vi "Actor Core.vi"(8 "error in":errorcluster, 11 "SongQueueActor in":refnum<class "SongQueueActor.lvclass">) -> (0 "error out":errorcluster, 3 "Actor out":refnum<class "Actor.lvclass">)   [LabVIEW 2015, in "SongQueueActor.lvlib" / "SongQueueActor.lvclass"]
doc: "(<B>Filename</B>: Actor Framework.lvlib:Actor.lvclass:Actor Core.vi)\n\nReceives messages to the actor, reacts to them, and initiates any error handling that may shut the actor down.\n\nDescendant classes may override this VI to append parallel tasks for the actor to complete while it handles messages. Overrides use the Call Parent Method node."
uses:
  SongQueueActor.lvclass
  <vilib>/ActorFramework/Actor/Actor.lvclass
  builds/xctls/Song Queue/Song Queue.lvlibp/app/xctls/SongQueue/Song Queue.xctl
  SongPlayerActor/SongPlayerActor/SongPlayerActor.lvclass
  builds/xctls/Song Queue/Song Queue.lvlibp/app/controls/Queue Song Display.ctl
  builds/xctls/Song Queue/Song Queue.lvlibp/file/MusicElement/Song/Song Duration.ctl
  builds/xctls/Song Queue/Song Queue.lvlibp/app/controls/Dequeue Control.ctl
  SongQueueActor.lvclass/SongQueueActor.ctl
  <vilib>/ActorFramework/Actor/Actor.lvclass/Actor.ctl
  <vilib>/ActorFramework/Message Enqueuer/Message Enqueuer.lvclass/Message Enqueuer.ctl
  <vilib>/ActorFramework/Message Enqueuer/Init from Existing Queue.vi
  <vilib>/ActorFramework/Message Enqueuer/Enqueue.vi
  <vilib>/ActorFramework/Message Priority Queue/Priority Enqueue.vi
  <vilib>/ActorFramework/Message Enqueuer/Message Enqueuer.lvclass
  <vilib>/ActorFramework/Stop Msg/Stop Msg.lvclass
  SongPlayerActor/SongPlayerActor Messages/Embed Actor Core In Subpanel Msg/Embed Actor Core In Subpanel Msg.lvclass
  builds/xctls/Song Queue/Song Queue.lvlibp
  builds/xctls/Song Queue/Song Queue.lvlibp/file/MusicElement/Song/Song.lvclass
  SongQueueActor Messages/Remove Song From Queue by Index Msg/Remove Song From Queue by Index Msg.lvclass
panel:
  in  "UI Tabs":enum32{"Main", "Debug"}(tab)
  in  "Song Queue":T1[](xcontrol)
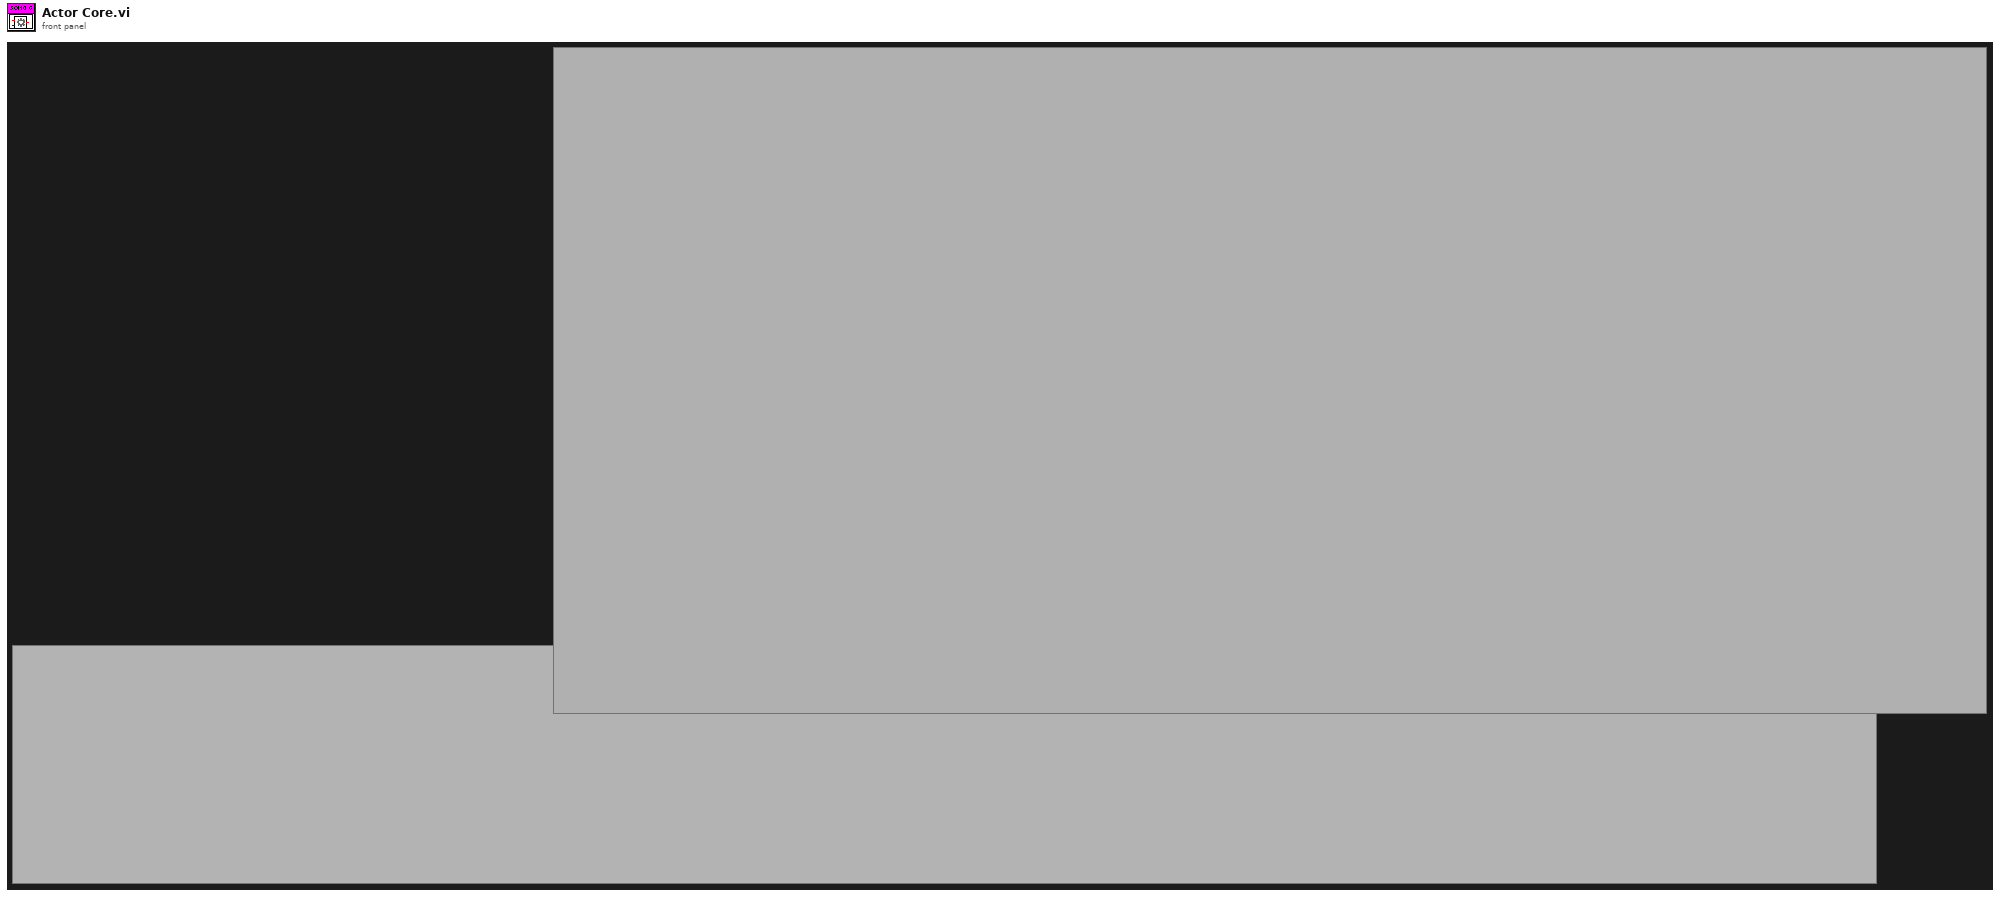
[diagram p1: front panel]
types:
  T1 = typedef "Song Queue.lvlibp/Queue Song Display.ctl" = cluster{"Song Name":string, "Artist":string, "Album":string, "Duration (s)":T2, "UID":string, "Dequeue":T3}
  T2 = typedef "Song Queue.lvlibp/Song.lvclass/Song Duration.ctl" = timestamp
  T3 = typedef "Song Queue.lvlibp/Dequeue Control.ctl" = bool
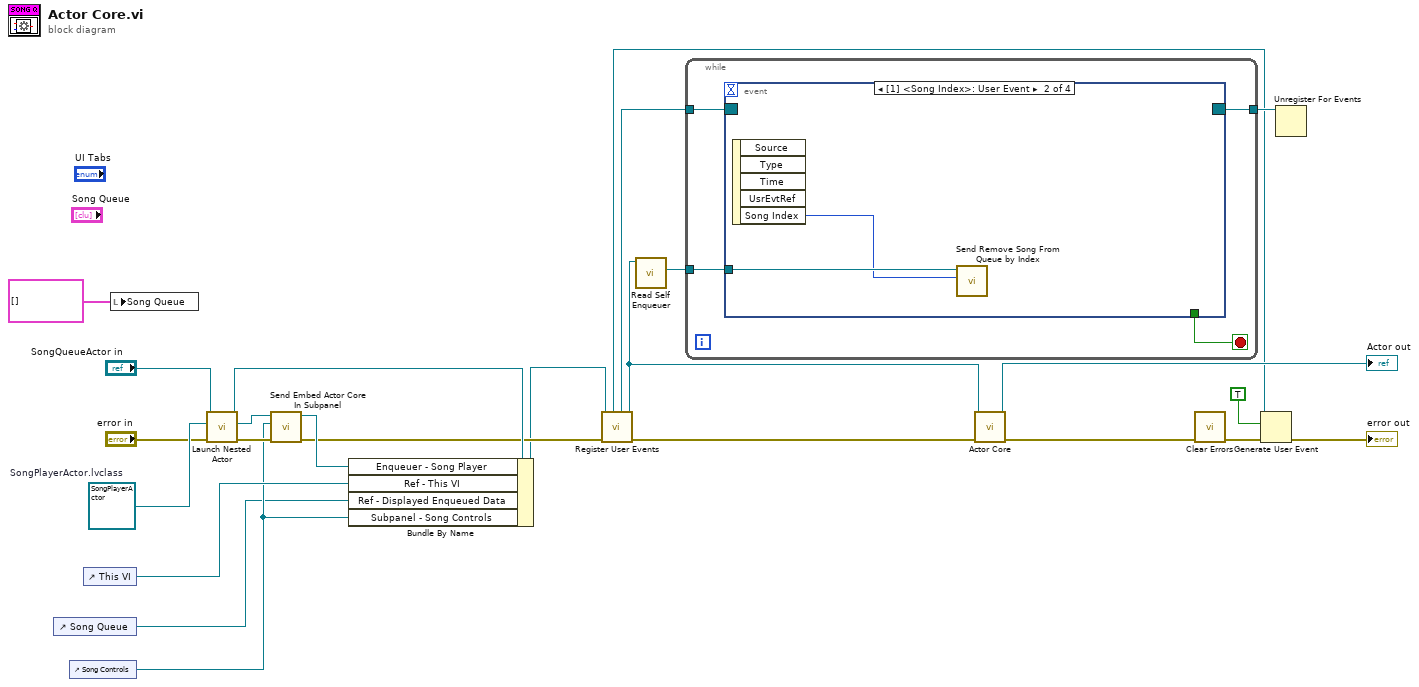
[diagram p0: block diagram]
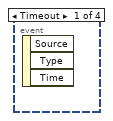
[diagram p2: hidden frame]
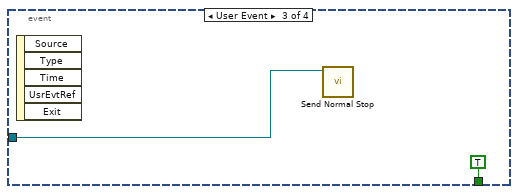
[diagram p3: hidden frame]
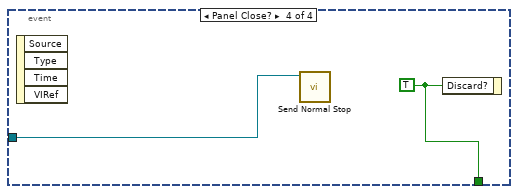
[diagram p4: hidden frame]
diagram:
  w17 = refnum<class "SongPlayerActor.lvclass"> refnum  # SongPlayerActor.lvclass
  n1 = control-ref of="Song Queue"() -> (w8:refnum<vi>)
  n2 = control-ref of="Song Controls"() -> (w10:refnum<vi>)
  n3 = control-ref of="This VI"() -> (w11:refnum<vi>)
  n4 = local write "Song Queue"(T1[] [] ("Song Queue")) -> ()
  n5 = call <vilib>:"Launch Nested Actor.vi"("error in (no error)"="error in", "Nested Actor"=w17, "Caller Actor in"="SongQueueActor in") -> ("error out"=w16:errorcluster, "Nested Actor's Enqueuer"=w15:refnum<class "Message Enqueuer.lvclass">, "Caller Actor out"=w12:refnum<class "SongQueueActor.lvclass">)  [unwired: 6 in]
  n6 = call "Send Embed Actor Core In Subpanel.vi"("error in (no error)"=w16, "Subpanel"=w10, "Message Enqueuer in"=w15) -> ("error out"=w6:errorcluster, "Message Enqueuer out"=w7:refnum<class "Message Enqueuer.lvclass">)  [unwired: 7 in]
  n7 = Bundle By Name(cluster=w12, "Enqueuer - Song Player"=w7, "Ref - This VI"=w11, "Ref - Displayed Enqueued Data"=w8, "Subpanel - Song Controls"=w10) -> (w4:refnum<class "SongQueueActor.lvclass">)
  n8 = call "Register User Events.vi"("error in (no error)"=w6, "SongQueueActor in"=w4) -> ("error out"=w1:errorcluster, "SongQueueActor out"=w5:refnum<class "SongQueueActor.lvclass">, "Event Registration Refnum"=w2:refnum<event-registration>, "Exit Event"=w3:refnum<user-event>)  [unwired: 6 in]
  n9 = call <vilib>:"Read Self Enqueuer.vi"("Actor"=w5) -> ("Self Enqueuer"=w20:refnum<class "Message Enqueuer.lvclass">)  [unwired: 10 in]
  n10 = while {
    tunnel: w2 -> [w25]
    tunnel: [w27] -> w24
    tunnel: w20 -> [w26]
    stop <- w28 stop-if-true
    n11 = event shown="[1] <Song Index>: User Event" {
      selector: w25 -> [_ _ _ _]
      dyn-events: [_ _ _ _] -> w27
      timeout: _ -> [_ _ _ _]
      tunnel: [_ _ TRUE ("Exit") w34] -> w28
      tunnel: w26 -> [_ w30 w31 w33]
      event Timeout {
        n12 = event-data() -> ()  [unwired: 1 in, 3 out]
      }
      event User Event {
        n13 = event-data() -> ("Song Index"=w29:u32)  [unwired: 1 in, 4 out]
        n14 = call "Send Remove Song From Queue by Index.vi"("Index"=w29, "Message Enqueuer in"=w30) -> ()  [unwired: 8 in, 2 out]
      }
      event User Event {
        n15 = event-data() -> ()  [unwired: 1 in, 5 out]
        n16 = call <vilib>:"Send Normal Stop.vi"("Message Enqueuer"=w31) -> ()  [unwired: 10 in, 1 out]
      }
      event Panel Close? {
        w34 = TRUE ("Discard?")
        n17 = event-data() -> ()  [unwired: 1 in, 4 out]
        n18 = call <vilib>:"Send Normal Stop.vi"("Message Enqueuer"=w33) -> ()  [unwired: 10 in, 1 out]
        n19 = event-data("Discard?"=w34) -> ()  [unwired: 1 in, 1 out]
      }
    }
  }
  n20 = call-parent "Actor Core.vi"("error in"=w1, "Actor in"=w5) -> ("error out"=w23:errorcluster, "Actor out"=→"Actor out":refnum<class "Actor.lvclass">)  [unwired: 8 in]
  n21 = call <vilib>:"Clear Errors.vi"("error in (no error)"=w23) -> ("error out"=w21:errorcluster)  [unwired: 5 in, 1 out]
  n22 = Generate User Event(user event=w3, event data cluster=TRUE ("event data"), error in=w21) -> (error out=→"error out":errorcluster)  [unwired: 1 in, 1 out]
  n23 = Unregister For Events(event registration refnum=w24) -> ()  [unwired: 1 in, 1 out]
